vi "OnDataChange.vi"(0 "DataLogger in":refnum<class "DataLogger.lvclass">, 1 "DataExchange":T1, 3 "error in (no error)":errorcluster) -> (7 "DataLogger out":refnum<class "DataLogger.lvclass">, 10 "error out":errorcluster)   [LabVIEW 2020, in "DataLogger.lvlib" / "DataLogger.lvclass"]
uses:
  DataLogger.lvclass
  Hardware Abstraction Layer/Component/Device/Device/DataExchange.ctl
  DataLogger.lvclass/DataLogger.ctl
  Hardware Abstraction Layer/Component/GenericActor/GenericActor/GenericController.lvclass
  Interface/DataListener/DataListener.lvclass
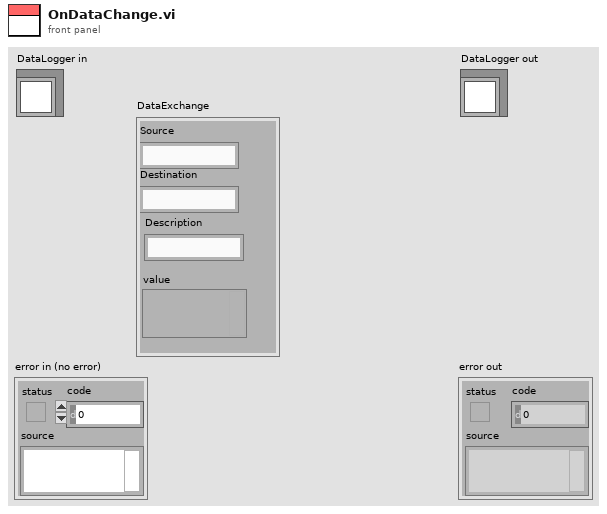
[diagram p1: front panel]
types:
  T1 = typedef "DataListener.lvclass/DataExchange.ctl" = cluster{"Source":string, "Destination":string, "Description":string, "value":variant}
  T2 = cluster{"StreamToDisk?":bool, "SingleStack?":bool, "Alert when finish?":bool, "TiffFileFullPath":path, "StreamFileFullPath":path}
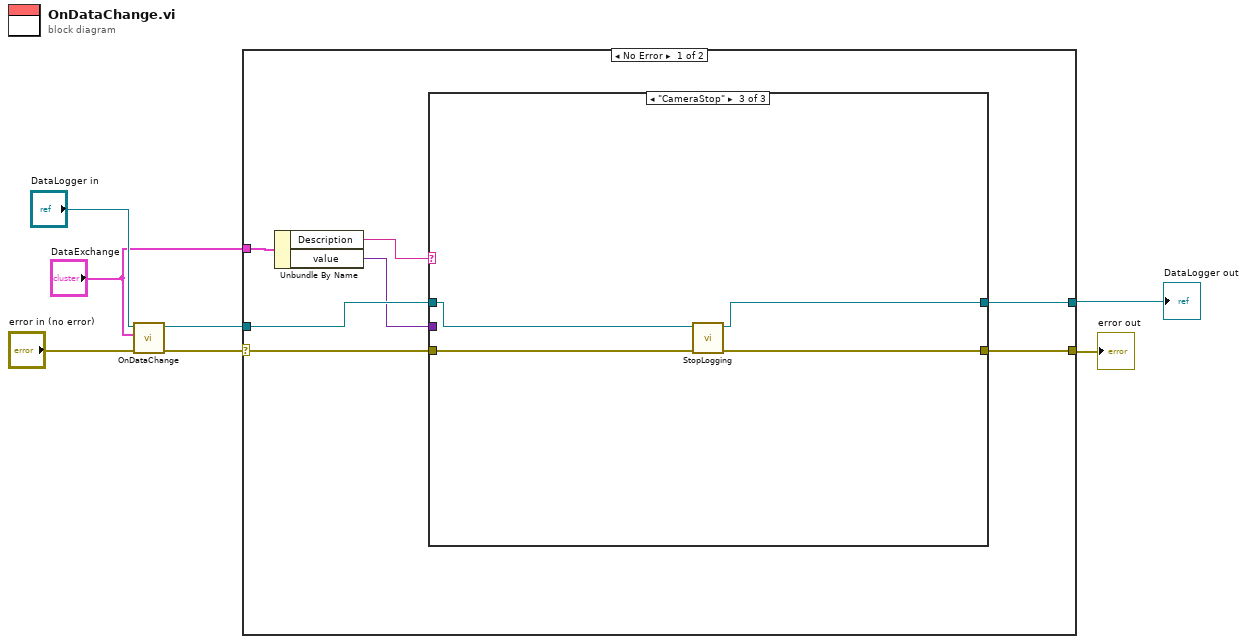
[diagram p0: block diagram]
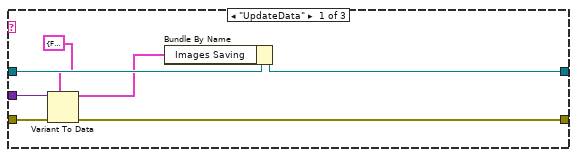
[diagram p2: hidden frame]
diagram:
  n1 = call-parent "OnDataChange.vi"("GRMActor in"="DataLogger in", "DataExchange"="DataExchange", "error in (no error)"="error in (no error)") -> ("GRMActor out"=w3:refnum<class "DataLogger.lvclass">, "error out"=w5:errorcluster)  [unwired: 6 in]
  n2 = case shown="No Error" w5 {
    selector: w5 -> [w10 w29]
    tunnel: [w9 w29] -> w4
    tunnel: w3 -> [w12 w28]
    tunnel: [w11 w28] -> w2
    tunnel: "DataExchange" -> [w14 _]
    frame No Error {
      n3 = Unbundle By Name(w14) -> ("Description"=w13:string, "value"=w8:variant)
      n4 = case shown="\"CameraStop\"" w13 {
        tunnel: w12 -> [w21 w23 w25]
        tunnel: [w19 w23 w24] -> w11
        tunnel: w10 -> [w20 w22 w27]
        tunnel: [w18 w22 w26] -> w9
        tunnel: w8 -> [w17 _ _]
        frame "UpdateData" {
          n5 = Variant To Data(error in=w20, type=T2 {"StreamToDisk?"=FALSE, "SingleStack?"=FALSE, "Alert when finish?"=FALSE, "TiffFileFullPath"=path "", "StreamFileFullPath"=path ""} ("Images Saving"), Variant=w17) -> (data=w15:T2, error out=w18:errorcluster)
          n6 = Bundle By Name(cluster=w21, "Images Saving"=w15) -> (w19:refnum<class "DataLogger.lvclass">)
        }
        frame Default {
        }
        frame "CameraStop" {
          n7 = call-dynamic "StopLogging.vi"("error in (no error)"=w27, "DataLogger in"=w25) -> ("error out"=w26:errorcluster, "DataLogger out"=w24:refnum<class "DataLogger.lvclass">)  [unwired: 8 in]
        }
      }
    }
    frame Error {
    }
  }
  "error out" <- w4
  "DataLogger out" <- w2
